vi "AnalogWrite.vi"(3 "error in (no error)":errorcluster, 4 "analogWrite":dbl(knob) scale=0.0..5.0, 6 "VISA Refnum in":refnum<visa-resource-name>) -> (0 "error out":errorcluster, 1 "Data Return":u8[](array[numeric]), 2 "VISA Refnum out":refnum<visa-resource-name>)   [LabVIEW 2016]
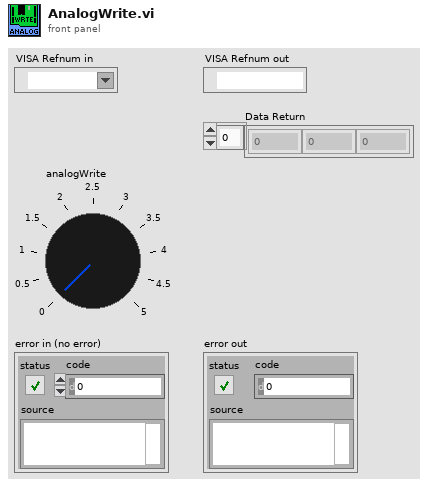
[diagram p1: front panel]
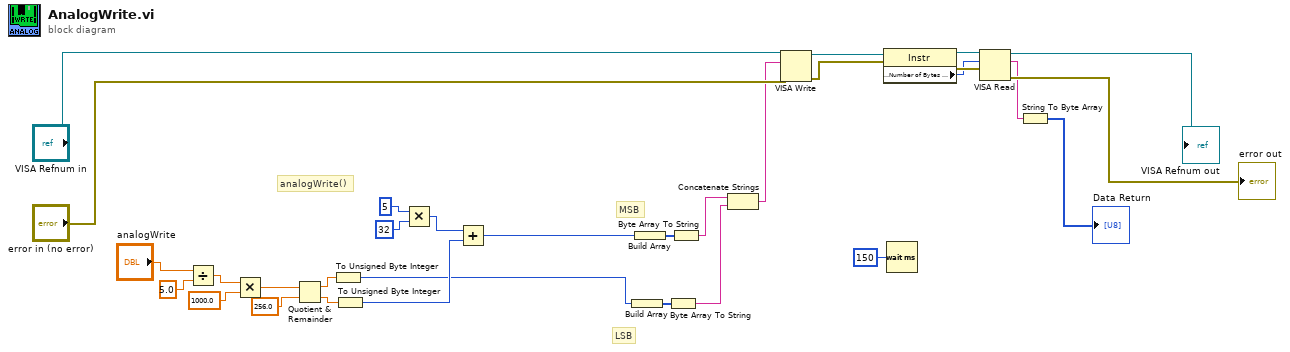
[diagram p0: block diagram]
diagram:
  # "LSB"
  # "MSB"
  # "analogWrite()"
  n1 = Divide(x="analogWrite", y=5.0) -> (x/y=w25:dbl)
  n2 = Multiply(x=w25, y=1000.0) -> (x*y=w27:dbl)
  n3 = Quotient & Remainder(x=w27, y=256.0) -> (x-y*floor(x/y)=w30:dbl, floor(x/y)=w29:dbl)
  n4 = To Unsigned Byte Integer(number=w30) -> (unsigned 8bit integer=w1:u8)
  n5 = To Unsigned Byte Integer(number=w29) -> (unsigned 8bit integer=w3:u8)
  n6 = Multiply(x=u8 5, y=u8 32) -> (x*y=w4:u8)
  n7 = Add(x=w4, y=w3) -> (x+y=w2:u8)
  n8 = Build Array(w1) -> (w21:u8[])
  n9 = Build Array(w2) -> (w13:u8[])
  n10 = Byte Array To String(unsigned byte array=w21) -> (string=w22:string)
  n11 = Byte Array To String(unsigned byte array=w13) -> (string=w14:string)
  n12 = Concatenate Strings(w14, w22) -> (w15:string)
  n13 = VISA Write(VISA resource name="VISA Refnum in", write buffer=w15, error in (no error)="error in (no error)") -> (VISA resource name out=w7:refnum<visa-resource-name>, error out=w6:errorcluster)  [unwired: 1 out]
  n14 = property class="Instr"(reference=w7, error in=w6) -> (reference out=w10:refnum<visa-resource-name>, error out=w9:errorcluster, "Serial Settings:Number of Bytes at Serial Port"=w8:u32)
  n15 = Wait (ms)(milliseconds to wait=u32 150) -> ()  [unwired: 1 out]
  n16 = VISA Read(VISA resource name=w10, byte count=w8, error in (no error)=w9) -> (VISA resource name out=→"VISA Refnum out":refnum<visa-resource-name>, read buffer=w16:string, error out=→"error out":errorcluster)  [unwired: 1 out]
  n17 = String To Byte Array(string=w16) -> (unsigned byte array=→"Data Return":u8[])
